vi "grab_image_topLvl_v02.vi"(8 "error in":errorcluster, 10 "orig image":T3, 11 "cam info in":T1={"camera type"=enum."Qcam", "cam handle"=0, "data handle"=0, "cam size"=[]}) -> (0 "error out":errorcluster, 2 "orig image out":T3, 3 "cam info out":T1={"camera type"=enum."Qcam", "cam handle"=0, "data handle"=0, "cam size"=[]})   [LabVIEW 2015]
uses:
  <vilib>/vision/Image Controls.llb/IMAQ Image.ctl
  controls/cam_info.ctl
  controls/cam_type-v02.ctl
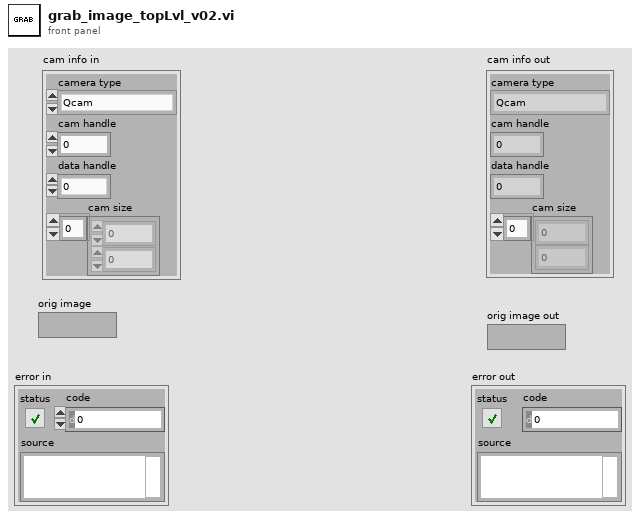
[diagram p1: front panel]
types:
  T1 = typedef "cam_info.ctl" = cluster{"camera type":T2, "cam handle":u32, "data handle":u32, "cam size":i32[]}
  T2 = typedef "cam_type-v02.ctl" = enum16{"HamamatsuORCA05G", "Qcam", "optiMOS"}
  T3 = typedef "IMAQ Image.ctl" = refnum<image>
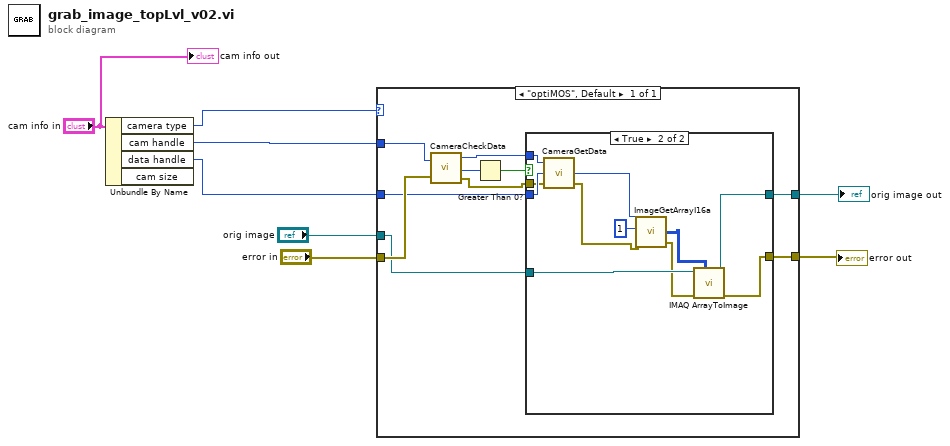
[diagram p0: block diagram]
diagram:
  n1 = Unbundle By Name("cam info in") -> ("camera type"=w3:T2, "cam handle"=w4:u32, "data handle"=w2:u32)  [unwired: 1 out]
  n2 = case shown="\"optiMOS\", Default" w3 {
    tunnel: w4 -> [w18]
    tunnel: "error in" -> [w17]
    tunnel: "orig image" -> [w10]
    tunnel: [w11] -> w6
    tunnel: [w9] -> w5
    tunnel: w2 -> [w14]
    frame "optiMOS", Default {
      n3 = call <userlib>:"CameraCheckData.vi"("Camera Handle"=w18, "error in"=w17) -> ("Camera Handle"=w13:u32, "Number Of Frames Available"=w16:i32, "error out"=w12:errorcluster)
      n4 = Greater Than 0?(x=w16) -> (x > 0?=w15:bool)
      n5 = case shown="True" w15 {
        tunnel: w14 -> [_ w31]
        tunnel: w13 -> [_ w30]
        tunnel: w12 -> [w19 w29]
        tunnel: [w19 w26] -> w11
        tunnel: w10 -> [w20 w28]
        tunnel: [w20 w27] -> w9
        frame False {
        }
        frame True {
          n6 = call <userlib>:"CameraGetData.vi"("error in"=w29, "Data Handle"=w31, "Camera Handle"=w30) -> ("error out"=w23:errorcluster, "Data Handle"=w25:u32)  [unwired: 1 out]
          n7 = call <userlib>:"ImageGetArrayI16a.vi"("error in (no error)"=w23, "Z Position"=u32 1 ("Z position"), "Data Handle"=w25) -> ("error out"=w22:errorcluster, "Array"=w21:i16[][])  [unwired: 1 in, 1 out]
          n8 = call "IMAQ ArrayToImage"("Image Pixels (U16)"=w21, "error in (no error)"=w22, "Image"=w28) -> ("error out"=w26:errorcluster, "Image Out"=w27:T3)  [unwired: 7 in]
        }
      }
    }
  }
  "error out" <- w6
  "orig image out" <- w5
  "cam info out" <- "cam info in"
